vi "Write BIU Configuration.vi"(8 "error in":errorcluster, 10 "biu configuration":T2, 11 "custom device ref":T1 format="%.0x") -> (0 "error out":errorcluster, 3 "custom device ref out":T1 format="%.0x")   [LabVIEW 2020, in "AIM MIL-STD-1553 Scripting.lvlib"]
doc: "Writes AIM MIL-STD 1553 BIU configuration information provided in the input cluster, including: Major Frames, Minor Frames, Acyclic Frames, Terminal Names/Addresses, Messages, and the Port number (also called hardware channel)."
uses:
  AIM MIL-STD-1553 Scripting.lvlib
  <vilib>/NI VeriStand/Custom Device API/Custom Device Item Ref.ctl
  Shared/1553 Channel.ctl
  Shared/Address.ctl
  Shared/Major Frame Definition.ctl
  Shared/Minor Frame Definition.ctl
  Shared/Message Definition.ctl
  Shared/Message Type.ctl
  Shared/Terminal Endpoint.ctl
  Shared/Parameter Definition.ctl
  <vilib>/NI VeriStand/Custom Device API/Custom Device API.lvlib
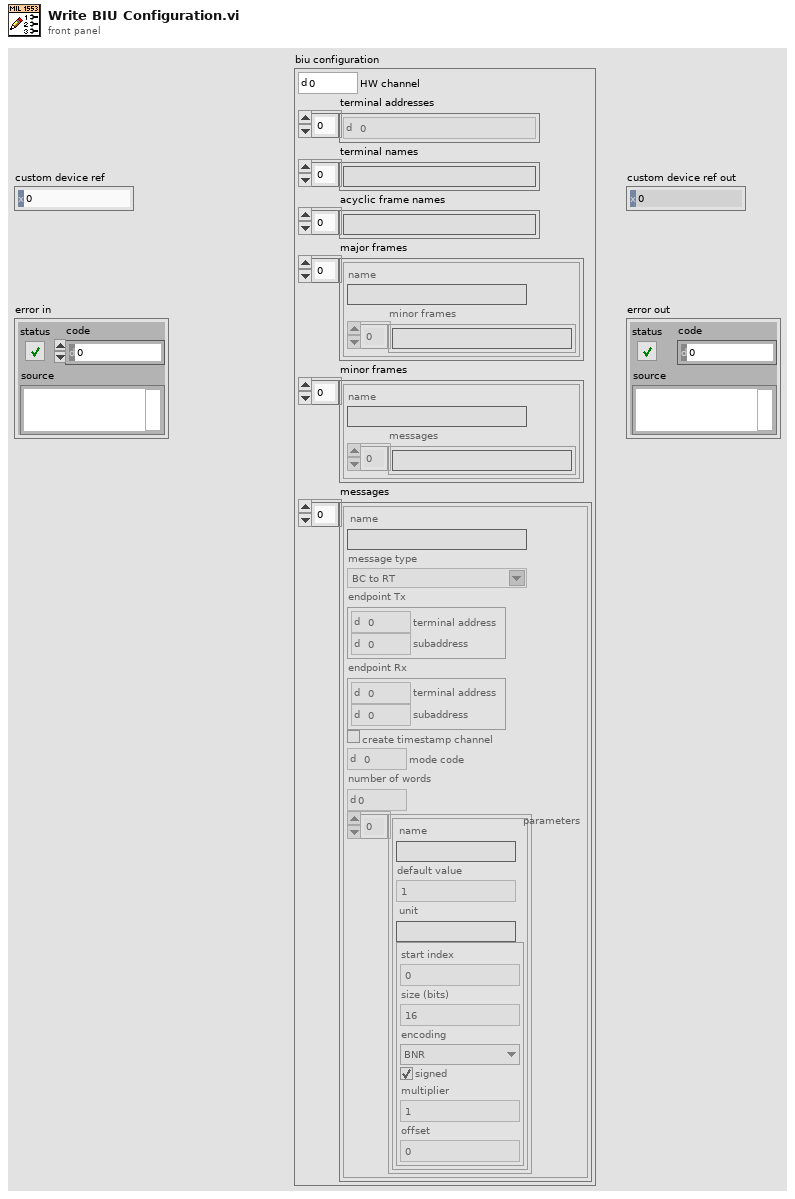
[diagram p1: front panel]
types:
  T1 = typedef "Custom Device API.lvlib/Custom Device Item Ref.ctl" = u64
  T2 = typedef "1553 Channel.ctl" = cluster{"HW channel":u16, "terminal addresses":T3[], "terminal names":string[], "acyclic frame names":string[], "major frames":T4[], "minor frames":T5[], "messages":T6[]}
  T3 = typedef "Address.ctl" = u16
  T4 = typedef "Major Frame Definition.ctl" = cluster{"name":string, "minor frames":string[]}
  T5 = typedef "Minor Frame Definition.ctl" = cluster{"name":string, "messages":string[]}
  T6 = typedef "Message Definition.ctl" = cluster{"name":string, "message type":T7, "endpoint Tx":T8, "endpoint Rx":T8, "create timestamp channel":bool, "mode code":u16, "number of words":u16, "parameters":cluster{"name":string, "default value":dbl, "unit":string, "parameter definition":T9}[]}
  T7 = typedef "Message Type.ctl" = string
  T8 = typedef "Terminal Endpoint.ctl" = cluster{"terminal address":T3, "subaddress":T3}
  T9 = typedef "Parameter Definition.ctl" = cluster{"start index":i32, "size (bits)":i32, "encoding":enum16{"BNR", "BCD", "Discrete"}, "signed":bool, "multiplier":dbl, "offset":dbl}
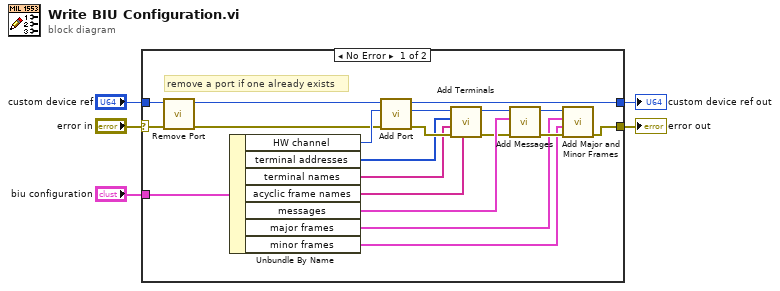
[diagram p0: block diagram]
diagram:
  n1 = case shown="No Error" "error in" {
    selector: "error in" -> [w8 w26]
    tunnel: [w25 w26] -> w5
    tunnel: [w24 w27] -> w4
    tunnel: "biu configuration" -> [w23 _]
    tunnel: "custom device ref" -> [w9 w27]
    frame No Error {
      # "remove a port if one already exists"
      n2 = call "Remove Port.vi"("error in"=w8, "custom device ref"=w9) -> ("error out"=w7:errorcluster, "custom device ref out"=w6:T1)  [unwired: 8 in]
      n3 = Unbundle By Name(w23) -> ("HW channel"=w22:u16, "terminal addresses"=w16:T3[], "terminal names"=w14:string[], "acyclic frame names"=w15:string[], "messages"=w21:T6[], "major frames"=w11:T4[], "minor frames"=w10:T5[])
      n4 = call "Add Port.vi"("error in"=w7, "port number"=w22, "custom device ref"=w6) -> ("error out"=w19:errorcluster, "port"=w20:T1, "custom device ref out"=w24:T1)  [unwired: 6 in]
      n5 = call "Add Terminals.vi"("acyclic frame names"=w15, "error in"=w19, "terminal names"=w14, "terminal addresses"=w16, "port in"=w20) -> ("error out"=w17:errorcluster, "port out"=w18:T1)  [unwired: 5 in]
      n6 = call "Add Messages.vi"("error in"=w17, "messages"=w21, "port in"=w18) -> ("error out"=w12:errorcluster, "port out"=w13:T1)  [unwired: 7 in]
      n7 = call "Add Major and Minor Frames.vi"("error in"=w12, "minor frames"=w10, "major frames"=w11, "port in"=w13) -> ("error out"=w25:errorcluster)  [unwired: 6 in, 1 out]
    }
    frame Error {
    }
  }
  "error out" <- w5
  "custom device ref out" <- w4
